vi "Structure Reporter.vi"() -> ()   [LabVIEW 2023, in "VIDoc Parsing.lvlib" / "Structure Reporter.lvlib"]
uses:
  Structure Reporter.lvlib
  UI Style.vi
panel:
  out "Tree":string(tree)
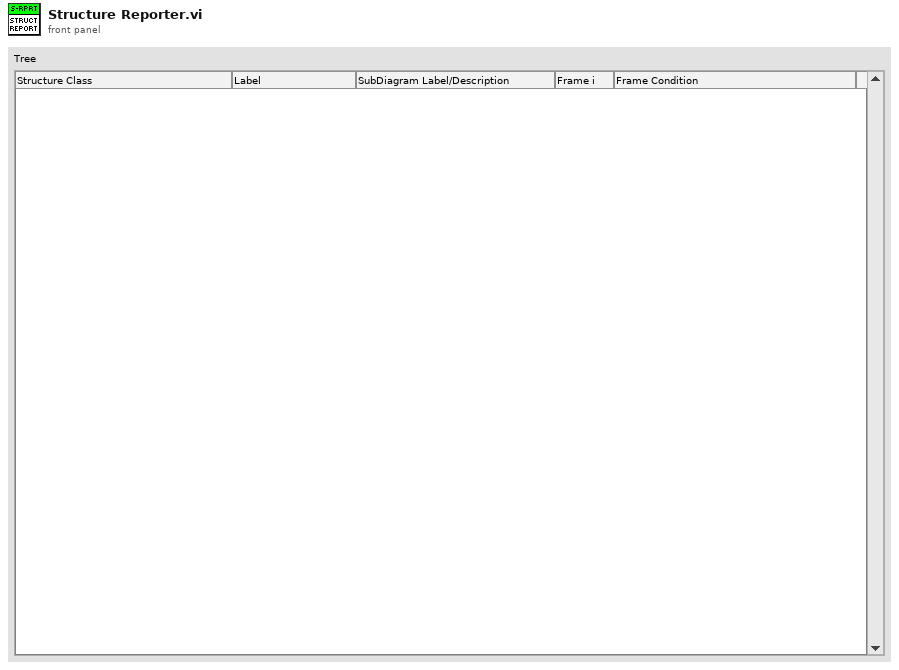
[diagram p1: front panel]
types:
  T1 = typedef "VIDoc Parsing.lvlib/Structure Reporter.lvlib/Structure Result 2.ctl" = cluster{"Depth":i32, "Top":i32, "Left":i32, "Frame index":i32, "Struct":i32, "Object Class Name":string, "Object UID":i32, "Label Visible":bool, "Object Label":string, "SD Label Visible":bool, "Object SD Label":string, "Frame Name":string, "Diag UID":i32, "Owner Class Name":string, "Owner UID":i32, "Diag Struct":i32[], "Parent Struct":i32, "Diag UIDs":i32[], "Tree Name":string, "Diag Ref":refnum<vi>, "Owner Classes":string[], "Owner":refnum<vi>, "Owner UIDs":i32[], "Tag Indent":i32, "Tag Value":i32, "Child Tag":string}
  T2 = typedef "VIDoc Parsing.lvlib/Structure Reporter.lvlib/Tree Cluster.ctl" = cluster{"Object Class Name":string, "Labels":string[], "Child Tag":string, "Item Indent":i32, "Child Only?":bool, "Glyph Index":i32}
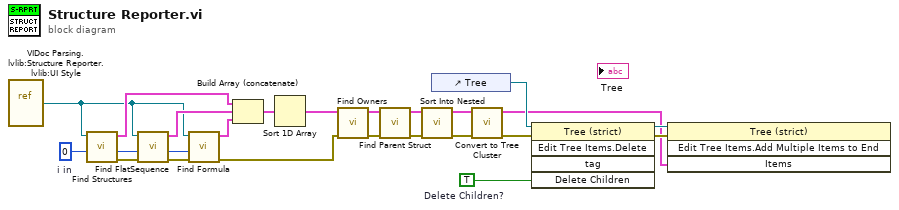
[diagram p0: block diagram]
diagram:
  w5 = TRUE  # Delete Children?
  w23 = 0  # i in
  n1 = vi-ref "VIDoc Parsing.lvlib:Structure Reporter.lvlib:UI Style.vi"() -> (w9:refnum<vi>)
  n2 = call "Find Structures.vi"("i in"=w23, "VI in"=w9) -> ("error out"=w15:errorcluster, "i out"=w22:i32, "Structures"=w24:T1[])  [unwired: 7 in]
  n3 = call "Find FlatSequence.vi"("error in (no error)"=w15, "i in"=w22, "VI in"=w9) -> ("error out"=w14:errorcluster, "i out"=w19:i32, "FlatSequences"=w21:T1[])  [unwired: 6 in]
  n4 = call "Find Formula.vi"("error in (no error)"=w14, "i in"=w19, "VI in"=w9) -> ("error out"=w13:errorcluster, "Array"=w20:T1[])  [unwired: 6 in, 1 out]
  n5 = Build Array (concatenate)(w24, w21, w20) -> (w18:T1[])
  n6 = Sort 1D Array(array=w18) -> (sorted array=w17:T1[])
  n7 = call "Find Owners.vi"("error in (no error)"=w13, "Array in"=w17) -> ("error out"=w12:errorcluster, "Array out"=w16:T1[])  [unwired: 8 in]
  n8 = call "Find Parent Struct.vi"("error in (no error)"=w12, "Objects in"=w16) -> ("error out"=w10:errorcluster, "Found Parent Struct"=w11:T1[])  [unwired: 8 in]
  n9 = call "Sort Into Nested.vi"("error in (no error)"=w10, "Found Parent Struct"=w11) -> ("error out"=w8:errorcluster, "Nested Structures"=w7:T1[])  [unwired: 8 in]
  n10 = control-ref of="Tree"() -> (w3:refnum<vi>)
  n11 = call "Convert to Tree Cluster.vi"("error in (no error)"=w8, "Array in"=w7) -> ("error out"=w4:errorcluster, "Array out"=w1:T2[])  [unwired: 8 in]
  n12 = invoke class="Tree (strict)" method="Edit Tree Items.Delete"(reference=w3, error in=w4, "Delete Children"=w5) -> (reference out=w2:refnum<vi>, error out=w6:errorcluster)  [unwired: 2 in, 3 out]
  n13 = invoke class="Tree (strict)" method="Edit Tree Items.Add Multiple Items to End"(reference=w2, error in=w6, "Items"=w1) -> ()  [unwired: 1 in, 4 out]
